vi "ReadNet_Tensorflow.vi"(8 "error in":errorcluster, 10 "ConfigPath":path, 11 "ModelPath":path) -> (0 "error out":errorcluster, 3 "NET":refnum<class "NET.lvclass">)   [LabVIEW 2020, in "OpenLvVision_OpenCv.lvlib"]
doc: "Reads a network model stored in TensorFlow framework's format."
uses:
  OpenLvVision_OpenCv.lvlib
  NET/NET.lvclass
  _LvHelpers/EdvrObject/TypeDef/Edvr.ctl
  _LvHelpers/EdvrObject/EdvrObject.lvclass
  Dlls/OlvOpenCvWrapper.dll
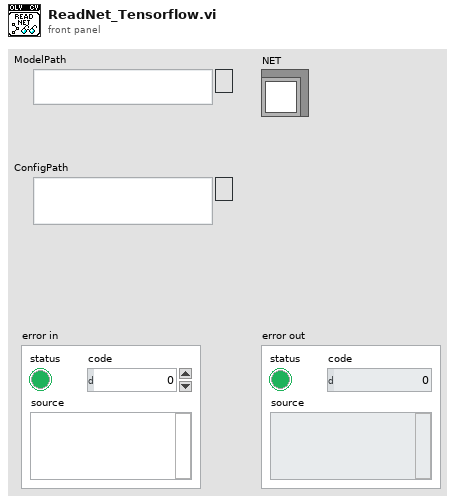
[diagram p1: front panel]
types:
  T1 = typedef "OpenLvVision_OpenCv.lvlib/EdvrObject.lvclass/Edvr.ctl" = refnum<data-value>
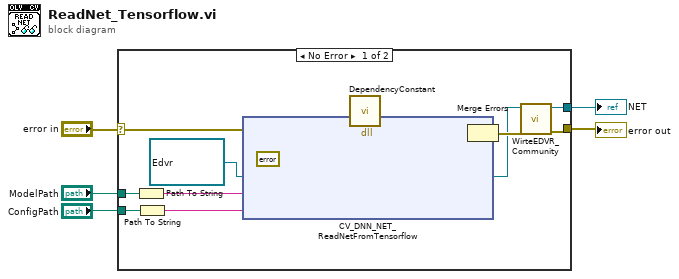
[diagram p0: block diagram]
diagram:
  n1 = case shown="No Error" "error in" {
    selector: "error in" -> [w15 w19]
    tunnel: [w13 w19] -> w4
    tunnel: [w11 _] -> w3
    tunnel: "ModelPath" -> [w10 _]
    tunnel: "ConfigPath" -> [w8 _]
    frame No Error {
      n2 = Path To String(path=w10) -> (string=w9:string)
      n3 = Path To String(path=w8) -> (string=w7:string)
      n4 = dll-call lib="C:/Users/lukas/Downloads/OpenLvVision_OpenCv/SourceCode/LabView/OpenLvVision_OpenCv/Dlls/OlvOpenCvWrapper.dll" fn="CV_DNN_NET_ReadNetFromTensorflow"(error in=w15, "Error"=errorcluster {"status"=FALSE, "code"=0, "source"=""} ("error out"), "edvrRef"=T1 refnum ("Edvr"), "modelPath"=w9, "configPath"=w7) -> (error out=w18:errorcluster, "Error"=w17:errorcluster, "edvrRef"=w12:T1)  [unwired: 5 in, 1 out]
      n5 = call "DependencyConstant.vi"() -> ()  [unwired: 12 in]
      n6 = Merge Errors(w18, w17) -> (w14:errorcluster)
      n7 = call "WirteEDVR_Community.vi"("error in"=w14, "Edvr"=w12) -> ("error out"=w13:errorcluster, "NET"=w11:refnum<class "NET.lvclass">)  [unwired: 8 in]
    }
    frame Error {
    }
  }
  "NET" <- w3
  "error out" <- w4
